vi "Messdaten_Periode.vi"(7 "Quelle Indices (Erzeugen=1, Extern=0)":bool=TRUE, 8 "error in":errorcluster, 10 "Messdaten_Indices_Extern":dbl[](array[numeric]), 11 "Messdaten_Eingang(1-D)":dbl[](array[numeric])) -> (0 "error out":errorcluster, 1 "Anzahl Messwerte":i32, 2 "Indices_der_Schwellwerte":dbl[](array[numeric]), 3 "Messdaten_einer_periode":dbl[](array[numeric]), 4 "max Messwert":dbl, 6 "min Messwert":dbl)   [LabVIEW 2016]
doc: "Dem Vi wird ein periodisches Signal in Form eines 1D-Arrays übergeben. Als Ausgabe Array wird das periodische Signal auf eine Periode reduziert.\n\nAnmerkung:\nPerdiodisches Signal muss x-Achsensymetrisch sein.\nÜber Boolschen Eingang kann zwischen Arbeiten mit selber erzeugten Periodenindices oder extern erzeugten Periodenindices umgeschaltet werden."
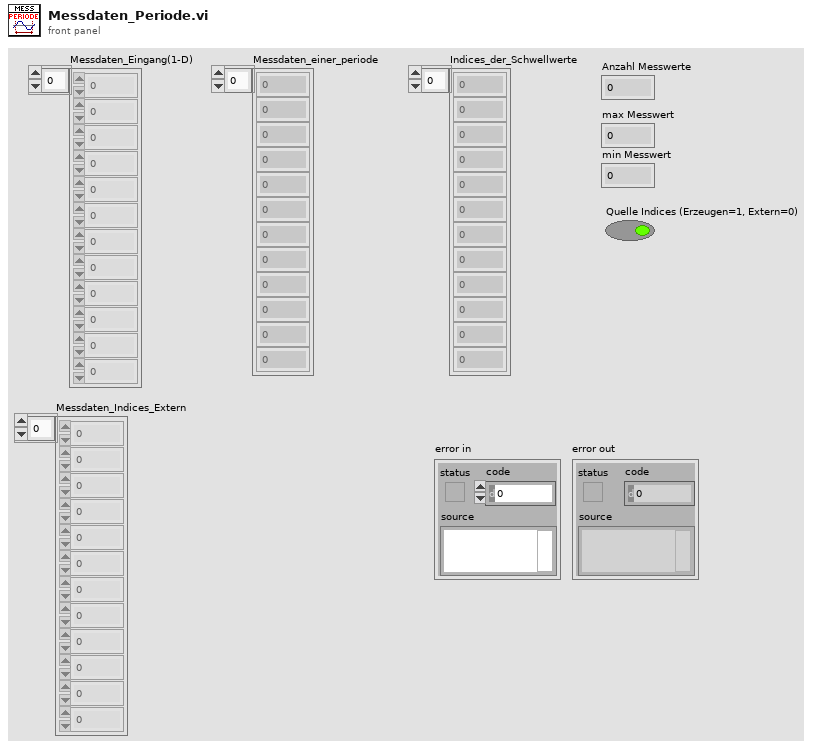
[diagram p1: front panel]
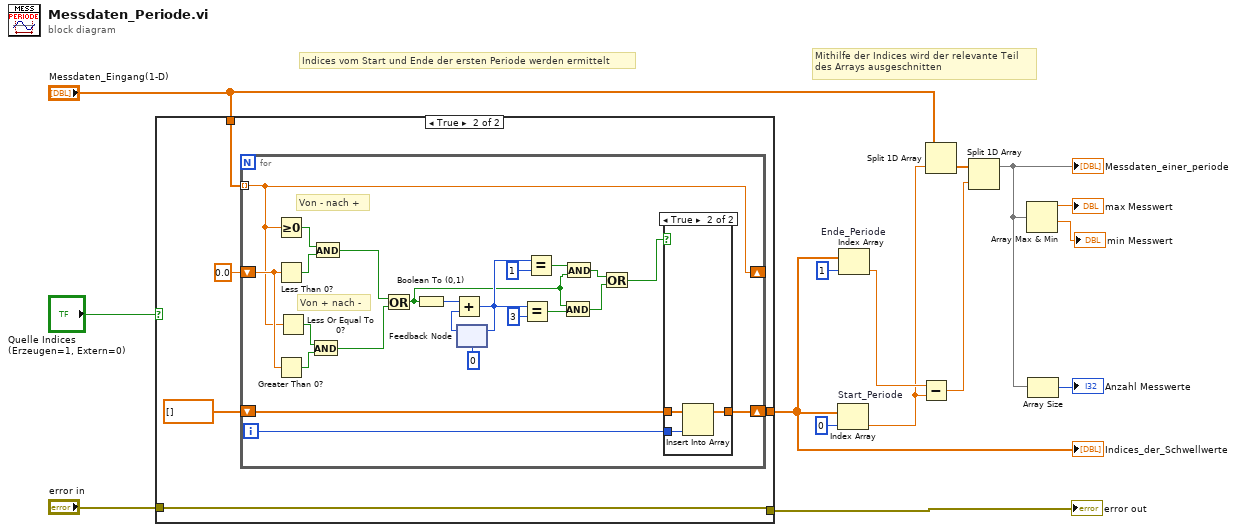
[diagram p0: block diagram]
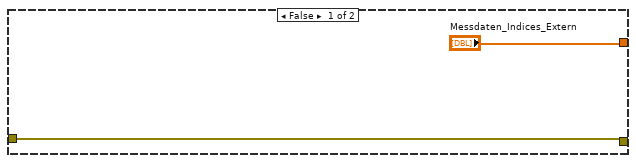
[diagram p2: hidden frame]
diagram:
  # "Mithilfe der Indices wird der relevante Teil\ndes Arrays ausgeschnitten"
  # "Indices vom Start und Ende der ersten Periode werden ermittelt"
  n1 = case shown="True" "Quelle Indices (Erzeugen=1, Extern=0)" {
    tunnel: ["Messdaten_Indices_Extern" w21] -> w13
    tunnel: "Messdaten_Eingang(1-D)" -> [_ w20]
    tunnel: [w16 w18] -> w2
    tunnel: "error in" -> [w16 w18]
    frame False {
    }
    frame True {
      n2 = for {
        tunnel: w20 -> [w38] mode=indexing
        shift-right: [w38] -> _
        shift-left: 0.0 ("element") -> [w39]
        shift-right: [w42] -> w21
        shift-left: dbl[] [] -> [w41]
        i -> [w43]
        # "Von + nach -"
        # "Von - nach +"
        n3 = Greater Or Equal To 0?(x=w38) -> (x >= 0?=w45:bool)
        n4 = Less Than 0?(x=w39) -> (x < 0?=w44:bool)
        n5 = Greater Than 0?(x=w39) -> (x > 0?=w37:bool)
        n6 = Less Or Equal To 0?(x=w38) -> (x <= 0?=w36:bool)
        n7 = And(x=w36, y=w37) -> (x .and. y?=w35:bool)
        n8 = And(x=w45, y=w44) -> (x .and. y?=w40:bool)
        n9 = Or(x=w40, y=w35) -> (x .or. y?=w23:bool)
        n10 = Boolean To (0,1)(Boolean=w23) -> (0, 1=w34:i16)
        n11 = feedback #1(i16 0) -> (w33:i16)
        n12 = Add(x=w34, y=w33) -> (x+y=w29:i16)
        n13 = feedback-in #1(w29) -> ()
        n14 = Equal?(x=w29, y=i16 3) -> (x = y?=w25:bool)
        n15 = Equal?(x=w29, y=i16 1) -> (x = y?=w27:bool)
        n16 = And(x=w23, y=w25) -> (x .and. y?=w24:bool)
        n17 = And(x=w27, y=w23) -> (x .and. y?=w26:bool)
        n18 = Or(x=w26, y=w24) -> (x .or. y?=w30:bool)
        n19 = case shown="True" w30 {
          tunnel: w43 -> [_ w47]
          tunnel: w41 -> [w46 w49]
          tunnel: [w46 w48] -> w42
          frame False {
          }
          frame True {
            n20 = Insert Into Array(array=w49, new element=w47) -> (w48:dbl[])  [unwired: 1 in]
          }
        }
      }
    }
  }
  "Indices_der_Schwellwerte" <- w13
  "error out" <- w2
  n21 = Index Array "Start_Periode"(array=w13, index=0) -> (element=w10:dbl)
  n22 = Index Array "Ende_Periode"(array=w13, index=1) -> (element=w11:dbl)
  n23 = Subtract(x=w11, y=w10) -> (x-y=w9:dbl)
  n24 = Split 1D Array(array="Messdaten_Eingang(1-D)", index=w10) -> (second subarray=w12:dbl[])  [unwired: 1 out]
  n25 = Split 1D Array(array=w12, index=w9) -> (first subarray=w7:dbl[])  [unwired: 1 out]
  "Messdaten_einer_periode" <- w7
  n26 = Array Max & Min(array=w7) -> (max value=→"max Messwert":dbl, min value=→"min Messwert":dbl)  [unwired: 2 out]
  n27 = Array Size(array=w7) -> (size(s)=→"Anzahl Messwerte":i32)
